vi "Test Initialize.vi"(0 "Test Template in":refnum<class "niDTS WLAN Rx Test.lvclass">, 11 "error in (no error)":errorcluster) -> (4 "Test Template out":refnum<class "niDTS WLAN Rx Test.lvclass">, 15 "error out":errorcluster)   [LabVIEW 2015, in "niDTS WLAN.lvlib" / "niDTS WLAN Rx Test.lvclass"]
uses:
  niDTS WLAN Rx Test.lvclass
  RiviInstDriver/niRfsgWlan/Objects/niRfsgWlan.lvclass
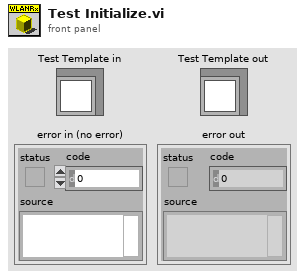
[diagram p1: front panel]
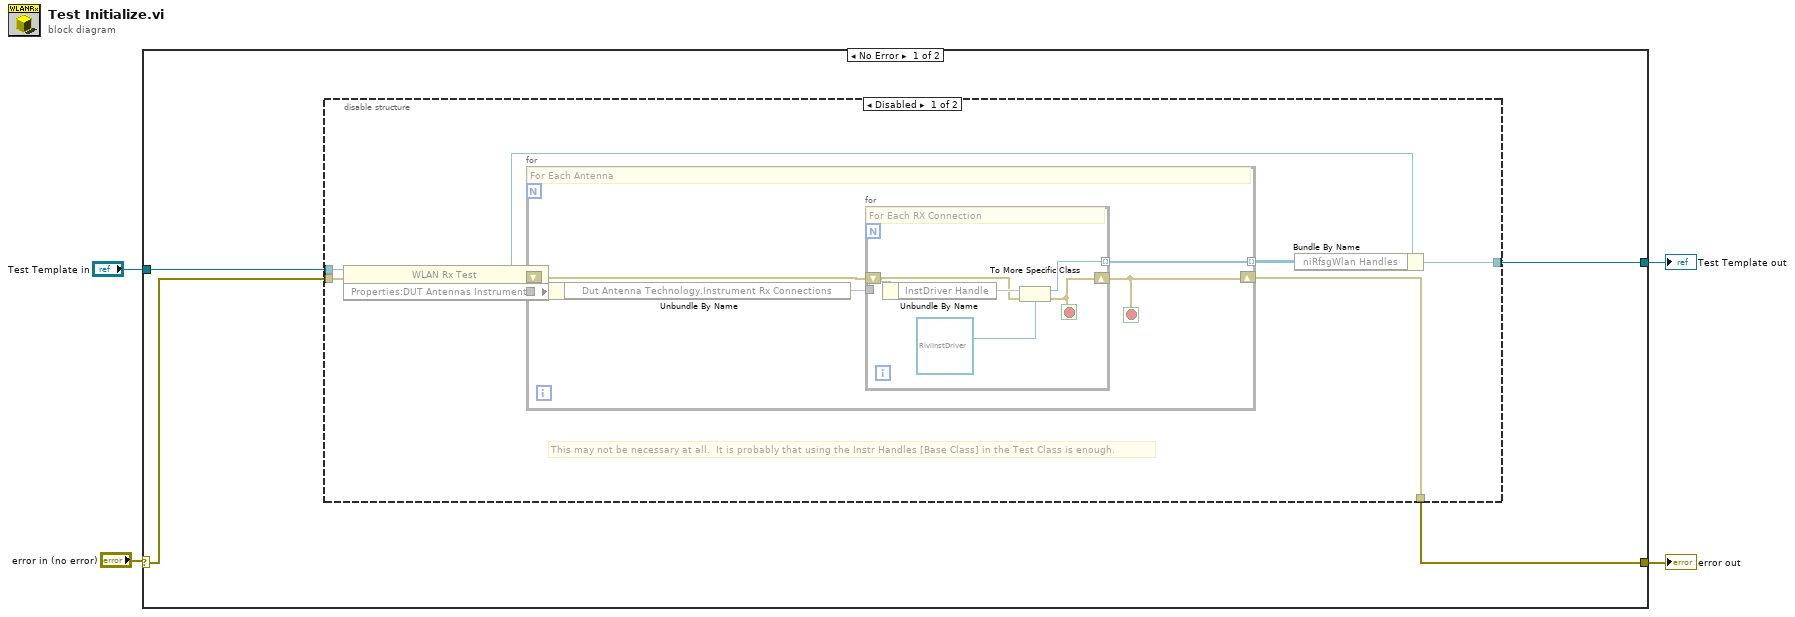
[diagram p0: block diagram]
diagram:
  n1 = case shown="No Error" "error in (no error)" {
    selector: "error in (no error)" -> [w7 w31]
    tunnel: [w5 w31] -> w3
    tunnel: [w6 w30] -> w1
    tunnel: "Test Template in" -> [w8 w30]
    frame No Error {
      n2 = disable-structure shown="Disabled" {
        disable-tunnel: w8 -> [w16 w29]
        disable-tunnel: w7 -> [w15 w28]
        disable-tunnel: [w10 w29] -> w6
        disable-tunnel: [w9 w28] -> w5
        frame Disabled {
          # "This may not be necessary at all.  It is probably that using the Instr Handles [Base Class] in the Test Class is enough."
          n3 = property class="WLAN Rx Test"(reference=w16, error in=w15) -> (reference out=w12:refnum<class "niDTS WLAN Rx Test.lvclass">, error out=w14:errorcluster, "Properties:DUT Antennas Instruments"=w13)
          n4 = for {
            tunnel: w13 -> [w21]
            shift-right: [w18] -> w9
            shift-left: w14 -> [w19]
            tunnel: [w17] -> w11 mode=indexing
            stop <- w18 stop-if-true
            # "For Each Antenna"
            n5 = Unbundle By Name(w21) -> ("Dut Antenna Technology.Instrument Rx Connections"=w20)
            n6 = for {
              tunnel: w20 -> [w27]
              shift-right: [w23] -> w18
              shift-left: w19 -> [w24]
              tunnel: [w22] -> w17 mode=indexing
              stop <- w23 stop-if-true
              # "For Each RX Connection"
              n7 = Unbundle By Name(w27) -> ("InstDriver Handle"=w26)
              n8 = To More Specific Class(target class=refnum<data-value> refnum ("RiviInstDriver Handle in"), reference=w26, error in=w24) -> (specific class reference=w22:refnum<data-value>, error out=w23:errorcluster)
            }
          }
          n9 = Bundle By Name(cluster=w12, "niRfsgWlan Handles"=w11) -> (w10:refnum<class "niDTS WLAN Rx Test.lvclass">)
        }
        frame Enabled {
        }
      }
    }
    frame Error {
    }
  }
  "error out" <- w3
  "Test Template out" <- w1
